vi "בדיקת מפל מתח בין הדקי הממסר תחת עומס bis5.vi"(8 "error":errorcluster, 10 "lines":tag="PXI1Slot8/port0/line1", 11 "Path for Log":path) -> (0 "error IO":errorcluster, 1 "בטוח כן/לא":bool, 2 "מפל מתח בין דקי הממסר תחת עומס":dbl, 3 "תוצאה זמנית":dbl)   [LabVIEW 2014]
uses:
  M9700 Driver/85/vi.lib/M9700 Modbus.llb/CTL Register Address.ctl
  M9700 Driver/86/vi.lib/M9700 Modbus.llb/CTL CMD Register.ctl
  <vilib>/Instr/_visa.llb/VISA Configure Serial Port (Instr).vi
  <vilib>/DAQmx/create/channels.llb/DAQmx Create Channel (DO-Digital Output).vi
  <vilib>/DAQmx/write.llb/DAQmx Write (Digital Bool 1Line 1Point).vi
panel:
  out "progress":dbl(slide) min=0.0 max=10.0 scale=0.0..10.0
  in  "stop":bool
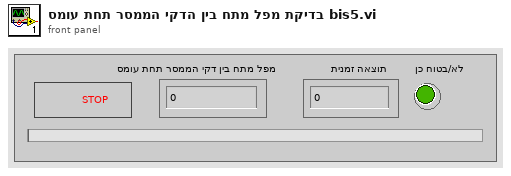
[diagram p1: front panel]
types:
  T1 = enum32{"Invalid", "Standard", "Closed", "Hidden", "Minimized", "Maximized"}
  T2 = typedef "CTL CMD Register.ctl" = u8
  T3 = typedef "CTL Register Address.ctl" = u16
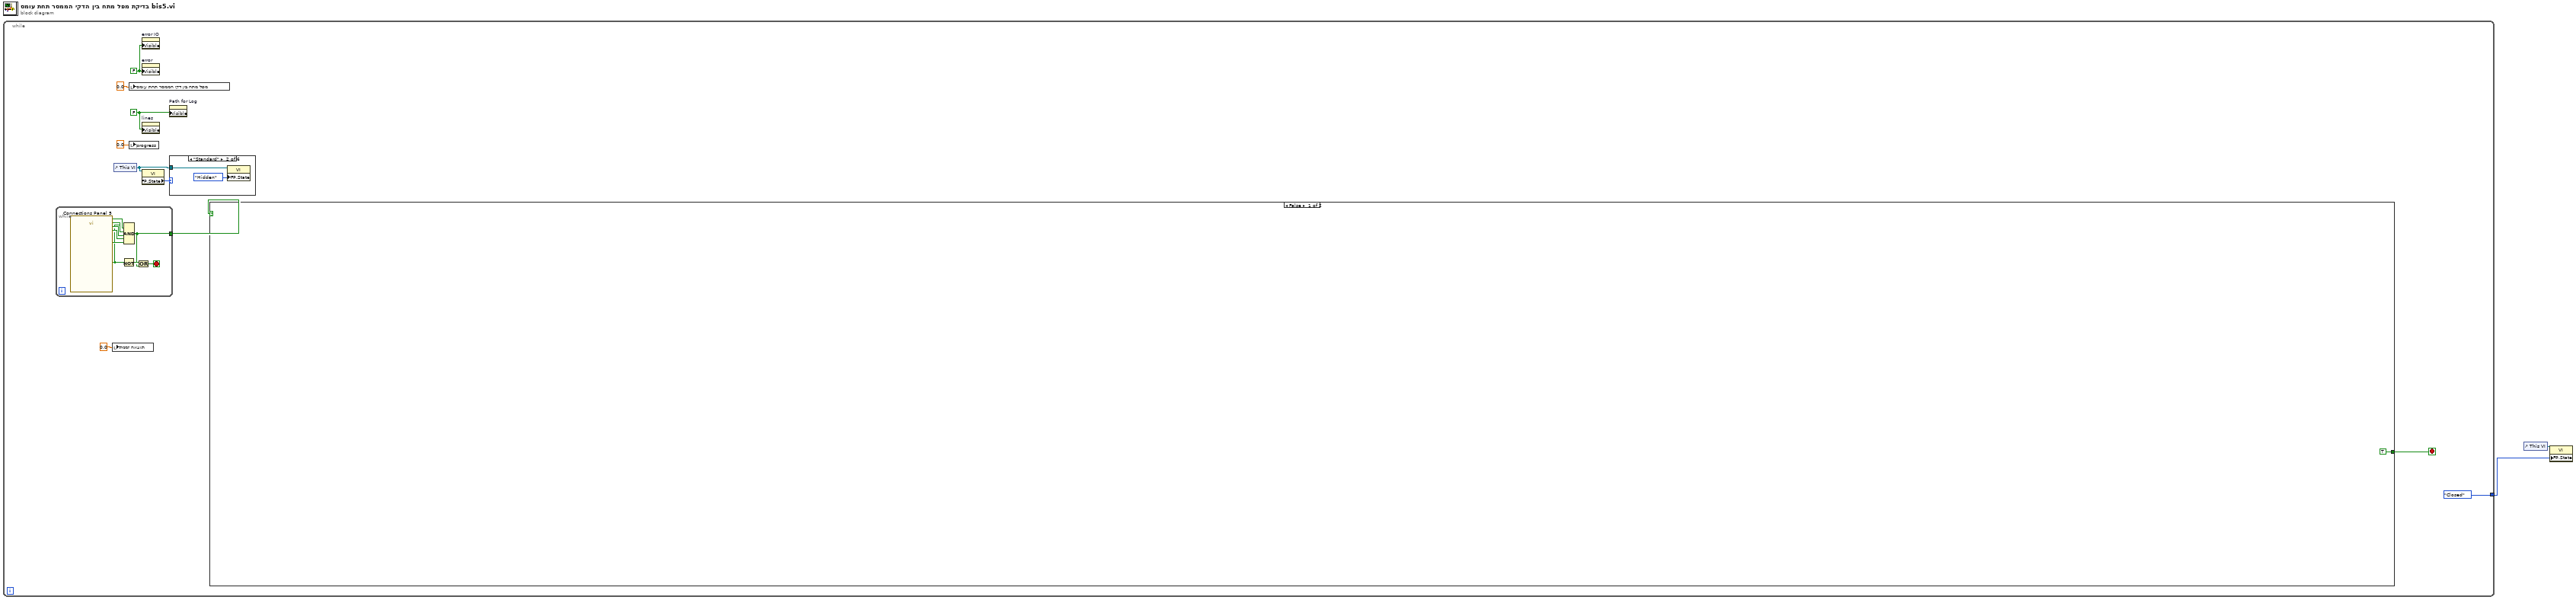
[diagram p0: block diagram]
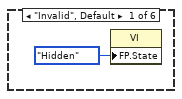
[diagram p2: hidden frame]
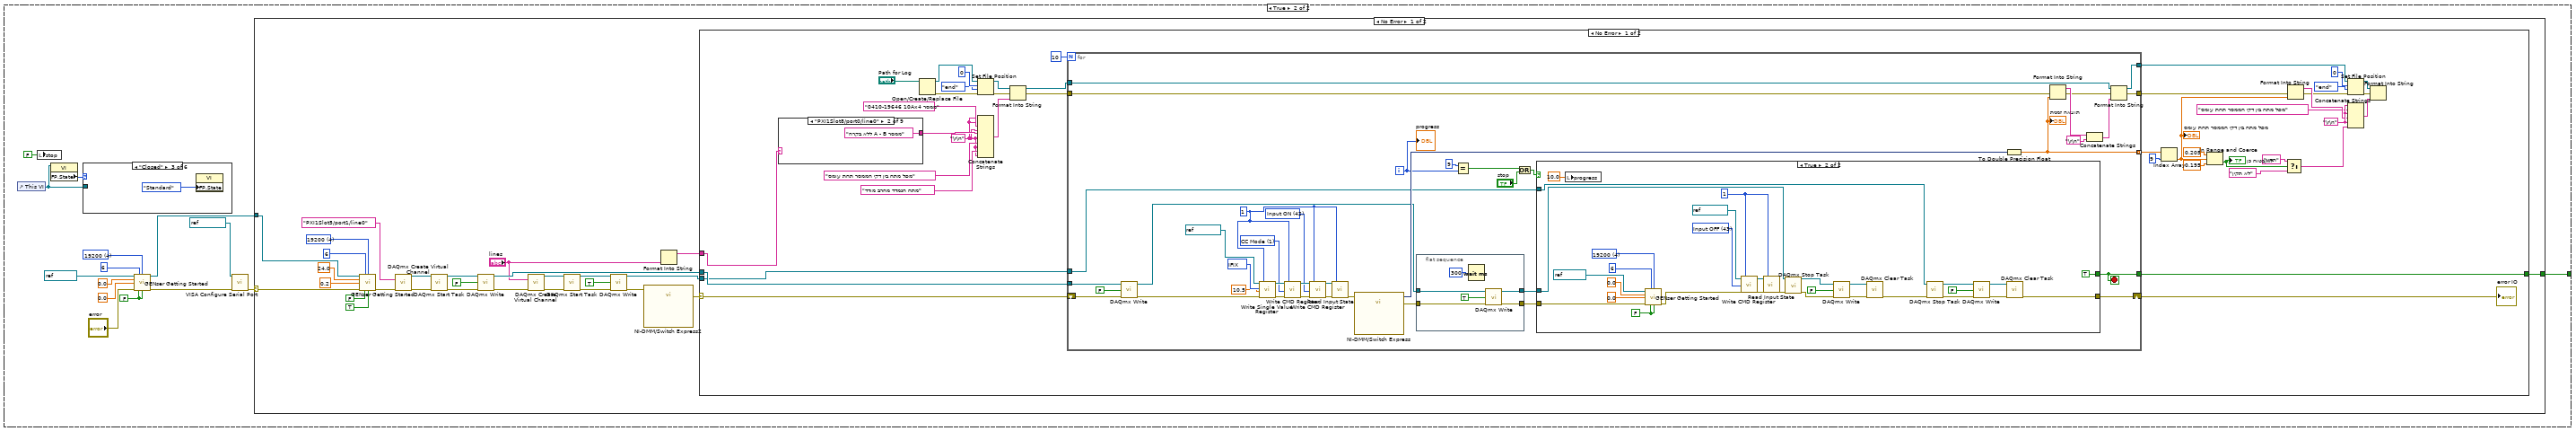
[diagram p7: hidden frame]
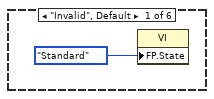
[diagram p8: hidden frame]
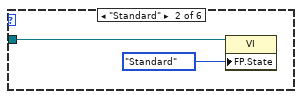
[diagram p9: hidden frame]
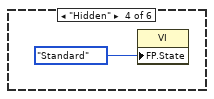
[diagram p10: hidden frame]
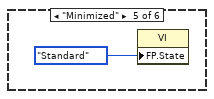
[diagram p11: hidden frame]
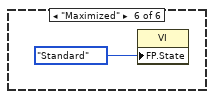
[diagram p12: hidden frame]
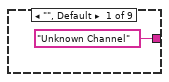
[diagram p13: hidden frame]
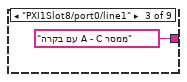
[diagram p14: hidden frame]
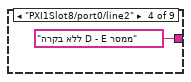
[diagram p15: hidden frame]
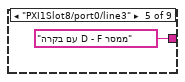
[diagram p16: hidden frame]
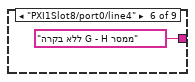
[diagram p17: hidden frame]
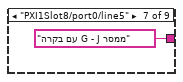
[diagram p18: hidden frame]
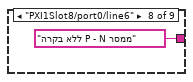
[diagram p19: hidden frame]
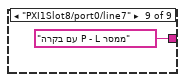
[diagram p20: hidden frame]
diagram:
  n1 = while {
    tunnel: [T1."Closed" ("Front Panel Window:State")] -> w1
    stop <- w12 stop-if-true
    w6 = FALSE ("Visible")
    w7 = FALSE ("Visible")
    n2 = while {
      tunnel: [w13] -> w11
      stop <- w16 stop-if-true
      n3 = call "Connections Panel 5.vi"() -> ("Input Name 10"=w17:bool, "Input Name 6"=w21:bool, "Input Name 7"=w20:bool, "Input Name 8"=w19:bool, "Input Name 9"=w18:bool, "OK"=w14:bool)  [unwired: 13 in, 1 out]
      n4 = Not(x=w14) -> (.not. x?=w15:bool)
      n5 = Compound Arithmetic op=AND(w14, w21, w20, w19, w18, w17) -> (w13:bool)
      n6 = Or(x=w15, y=w13) -> (x .or. y?=w16:bool)
    }
    n7 = local write "תוצאה זמנית"(0.0 ("תוצאה זמנית")) -> ()
    n8 = control-ref of="This VI"() -> (w5:refnum<vi>)
    n9 = local write "מפל מתח בין דקי הממסר תחת עומס"(0.0 ("מפל מתח בין דקי הממסר תחת עומס")) -> ()
    n10 = local write "progress"(0.0 ("progress")) -> ()
    n11 = property on="error IO" class="Clust (strict)"("Visible"=w7) -> ()  [unwired: 2 in, 2 out]
    n12 = property on="error" class="Clust (strict)"("Visible"=w7) -> ()  [unwired: 2 in, 2 out]
    n13 = property on="lines" class="DAQmxName"("Visible"=w6) -> ()  [unwired: 2 in, 2 out]
    n14 = property class="VI"(reference=w5) -> ("FP.State"=w4:T1)  [unwired: 1 in, 2 out]
    n15 = property on="Path for Log" class="Path"("Visible"=w6) -> ()  [unwired: 2 in, 2 out]
    n16 = case shown="\"Standard\"" w4 {
      tunnel: w5 -> [_ w23 _ _ _ _]
      frame "Invalid", Default {
        n17 = property class="VI"("FP.State"=T1."Hidden" ("Front Panel Window:State")) -> ()  [unwired: 2 in, 2 out]
      }
      frame "Standard" {
        n18 = property class="VI"(reference=w23, "FP.State"=T1."Hidden" ("Front Panel Window:State")) -> ()  [unwired: 1 in, 2 out]
      }
      frame "Closed" {
      }
      frame "Hidden" {
      }
      frame "Minimized" {
      }
      frame "Maximized" {
      }
    }
    n19 = case shown="False" w11 {
      tunnel: [TRUE w33] -> w12
      frame False {
      }
      frame True {
        w30 = FALSE ("Output On (T)")
        w37 = u16 4 items=["1200", "2400", "4800", "9600", "19200"] ("BAUD")
        n20 = control-ref of="This VI"() -> (w27:refnum<vi>)
        n21 = local write "stop"(FALSE ("stop")) -> ()
        n22 = property class="VI"(reference=w27) -> ("FP.State"=w28:T1)  [unwired: 1 in, 2 out]
        n23 = case shown="\"Closed\"" w28 {
          tunnel: w27 -> [_ w42 _ _ _ _]
          frame "Invalid", Default {
            n24 = property class="VI"("FP.State"=T1."Standard" ("Front Panel Window:State")) -> ()  [unwired: 2 in, 2 out]
          }
          frame "Standard" {
            n25 = property class="VI"(reference=w42, "FP.State"=T1."Standard" ("Front Panel Window:State")) -> ()  [unwired: 1 in, 2 out]
          }
          frame "Closed" {
            n26 = property class="VI"("FP.State"=T1."Standard" ("Front Panel Window:State")) -> ()  [unwired: 2 in, 2 out]
          }
          frame "Hidden" {
            n27 = property class="VI"("FP.State"=T1."Standard" ("Front Panel Window:State")) -> ()  [unwired: 2 in, 2 out]
          }
          frame "Minimized" {
            n28 = property class="VI"("FP.State"=T1."Standard" ("Front Panel Window:State")) -> ()  [unwired: 2 in, 2 out]
          }
          frame "Maximized" {
            n29 = property class="VI"("FP.State"=T1."Standard" ("Front Panel Window:State")) -> ()  [unwired: 2 in, 2 out]
          }
        }
        n30 = call "GENser Getting Started.vi"("VISA"=refnum<visa-resource-name> "COM6", "GEN Addr"=i16 6, "BAUD"=w37, "Voltage Limit"=0.0, "Current Limit"=0.0, "error"="error", "Reset (T)"=w30, "Output On (T)"=w30) -> ("VISA out"=w39:refnum<visa-resource-name>, "error out"=w26:errorcluster)  [unwired: 4 in, 2 out]
        n31 = call-poly "VISA Configure Serial Port"("VISA resource name"=refnum<visa-resource-name> "COM13", "error in (no error)"=w26) -> ("error out"=w31:errorcluster)  [unwired: 4 in, 9 out]
        n32 = case shown="No Error" w31 {
          selector: w31 -> [w73 _]
          tunnel: w39 -> [w75 _]
          tunnel: [w74 w209] -> w33
          frame No Error {
            w67 = u16 4 items=["1200", "2400", "4800", "9600", "19200"] ("BAUD")
            n33 = call "GENser Getting Started.vi"("VISA"=w75, "GEN Addr"=i16 6, "BAUD"=w67, "Voltage Limit"=24.0, "Current Limit"=0.2, "error"=w73, "Reset (T)"=FALSE, "Output On (T)"=TRUE) -> ("error out"=w61:errorcluster)  [unwired: 4 in, 3 out]
            n34 = call-poly <vilib>:"DAQmx Create Virtual Channel.vi"("lines"=tag "PXI1Slot5/port1/line0", "error in"=w61) -> ("task out"=w57:refnum<k21>, "error out"=w58:errorcluster)  [unwired: 12 in]
            n35 = call <vilib>:"DAQmx Start Task.vi"("task/channels in"=w57, "error in"=w58) -> ("task out"=w55:refnum<k21>, "error out"=w54:errorcluster)  [unwired: 12 in]
            n36 = call-poly <vilib>:"DAQmx Write.vi"("task/channels in"=w55, "data"=FALSE, "error in"=w54) -> ("task out"=w65:refnum<k21>, "error out"=w64:errorcluster)  [unwired: 10 in, 1 out]
            n37 = call-poly <vilib>:"DAQmx Create Virtual Channel.vi"("lines"="lines", "error in"=w64) -> ("task out"=w48:refnum<k21>, "error out"=w49:errorcluster)  [unwired: 12 in]
            n38 = call <vilib>:"DAQmx Start Task.vi"("task/channels in"=w48, "error in"=w49) -> ("task out"=w51:refnum<k21>, "error out"=w50:errorcluster)  [unwired: 12 in]
            n39 = call-poly <vilib>:"DAQmx Write.vi"("task/channels in"=w51, "data"=TRUE, "error in"=w50) -> ("task out"=w63:refnum<k21>, "error out"=w60:errorcluster)  [unwired: 10 in, 1 out]
            n40 = call "NI-DMM/Switch Express2"("error in"=w60) -> ("error out"=w59:errorcluster)  [unwired: 16 in, 2 out]
            n41 = Format Into String("lines") -> (resulting string=w66:string)  [unwired: 3 in, 1 out]
            n42 = case shown="No Error" w59 {
              selector: w59 -> [w117 _]
              tunnel: [w116 w204] -> w74
              tunnel: w65 -> [w115 _]
              tunnel: w66 -> [w114 _]
              tunnel: w63 -> [w113 _]
              frame No Error {
                w95 = "\r\n"
                w77 = "\r\n"
                n43 = case shown="\"PXI1Slot8/port0/line0\"" w114 {
                  tunnel: ["Unknown Channel" "ללא בקרה A - B ממסר" "עם בקרה A - C ממסר" "ללא בקרה D - E ממסר" "עם בקרה D - F ממסר" "ללא בקרה G - H ממסר" "עם בקרה G - J ממסר" "ללא בקרה P - N ממסר" "עם בקרה P - L ממסר"] -> w78
                  frame "", Default {
                  }
                  frame "PXI1Slot8/port0/line0" {
                  }
                  frame "PXI1Slot8/port0/line1" {
                  }
                  frame "PXI1Slot8/port0/line2" {
                  }
                  frame "PXI1Slot8/port0/line3" {
                  }
                  frame "PXI1Slot8/port0/line4" {
                  }
                  frame "PXI1Slot8/port0/line5" {
                  }
                  frame "PXI1Slot8/port0/line6" {
                  }
                  frame "PXI1Slot8/port0/line7" {
                  }
                }
                n44 = Open/Create/Replace File(file path (use dialog)="Path for Log") -> (refnum out=w105:refnum<file>, error out=w104:errorcluster)  [unwired: 5 in, 1 out]
                n45 = Set File Position(offset (in bytes) (0)=i64 0, refnum=w105, from (0:start)=enum16{"start", "end", "current"}."end", error in=w104) -> (refnum out=w101:refnum<file>, error out=w98:errorcluster)
                n46 = Concatenate Strings(w77, w77, "0410-19646 10Ax4 ממסר", w77, w78, w77, "מפל מתח בין דקי הממסר תחת עומס", w77, "מתח הנמדד מהרב מודד", w77) -> (w103:string)
                n47 = Format Into String(initial string=w101, error in=w98, w103) -> (resulting string=w96:refnum<file>, error out=w97:errorcluster)  [unwired: 1 in]
                n48 = for {
                  N: 10 -> [_]
                  tunnel: [w148] -> w116
                  shift-right: [w146] -> w76
                  shift-left: w117 -> [w141]
                  tunnel: [w128] -> w111 mode=indexing
                  tunnel: w115 -> [w142]
                  tunnel: w97 -> [w132]
                  tunnel: w96 -> [w134]
                  tunnel: [w131] -> w89
                  tunnel: [w130] -> w80
                  tunnel: w113 -> [w129]
                  i -> [w145]
                  stop <- w148 stop-if-true
                  w156 = T2 42 items=["CC Mode"=1, "CV Mode"=2, "CW Mode"=3, "CR Mode"=4, "Short Mode"=26, "Set SysPara"=41, "Input ON"=42, "Input OFF"=43] ("CMD Register Value")
                  w159 = u8 1 ("Load Address")
                  w162 = T2 1 items=["CC Mode"=1, "CV Mode"=2, "CW Mode"=3, "CR Mode"=4, "Short Mode"=26, "Set SysPara"=41, "Input ON"=42, "Input OFF"=43] ("CMD Register Value")
                  w165 = T3 2561 items=["REMOTE"=1283, "ISTATE"=1296, "CMD"=2560, "IFIX"=2561, "UFIX"=2563, "PFIX"=2565, "RFIX"=2567, "IMAX"=2612, "UMAX"=2614, "PMAX"=2616, "U"=2816, "I"=2818, "MODEL"=2822, "EDITION"=2823] ("Register Address")
                  n49 = call-poly <vilib>:"DAQmx Write.vi"("task/channels in"=w142, "data"=FALSE, "error in"=w141) -> ("task out"=w140:refnum<k21>, "error out"=w127:errorcluster)  [unwired: 10 in, 1 out]
                  n50 = call "Write Single Value Register.vi"("VISA resource name"=refnum<visa-resource-name> "COM13", "Starting Address(HEX)"=w165, "Register Single Value"=sgl 10.5, "error in"=w127, "Load Address"=w159) -> ("VISA resource name out"=w164:refnum<visa-resource-name>, "error out"=w163:errorcluster)  [unwired: 13 out]
                  n51 = call "Write CMD Register.vi"("VISA resource name"=w164, "CMD Value"=w162, "error in"=w163, "Load Address"=w159) -> ("VISA resource name out"=w160:refnum<visa-resource-name>, "error out"=w157:errorcluster)  [unwired: 14 out]
                  n52 = call "Write CMD Register.vi"("VISA resource name"=w160, "CMD Value"=w156, "error in"=w157, "Load Address"=w159) -> ("VISA resource name out"=w158:refnum<visa-resource-name>, "error out"=w155:errorcluster)  [unwired: 14 out]
                  n53 = call "Read Input State.vi"("VISA resource name"=w158, "error in"=w155, "Load Address"=w159) -> ("error out"=w154:errorcluster)  [unwired: 16 out]
                  n54 = call "NI-DMM/Switch Express"("error in"=w154) -> ("signals out"=w153:dynamicdata, "error out"=w143:errorcluster)  [unwired: 16 in, 1 out]
                  n55 = flat-sequence {
                    tunnel: [w171] -> w144
                    tunnel: w143 -> [w170]
                    tunnel: w140 -> [w168]
                    tunnel: [w167] -> w138
                    frame #0 {
                      n56 = Wait (ms)(milliseconds to wait=u32 300) -> ()  [unwired: 1 out]
                      n57 = call-poly <vilib>:"DAQmx Write.vi"("task/channels in"=w168, "data"=TRUE, "error in"=w170) -> ("task out"=w167:refnum<k21>, "error out"=w171:errorcluster)  [unwired: 10 in, 1 out]
                    }
                  }
                  n58 = Equal?(x=9, y=w145) -> (x = y?=w150:bool)
                  n59 = Or(x=w150, y="stop") -> (x .or. y?=w151:bool)
                  n60 = case shown="True" w151 {
                    tunnel: [FALSE TRUE] -> w148
                    tunnel: w144 -> [w172 w197]
                    tunnel: [w172 w177] -> w146
                    tunnel: w138 -> [_ w183]
                    tunnel: w129 -> [_ w175]
                    frame False {
                    }
                    frame True {
                      w191 = u8 1 ("Load Address")
                      w194 = T2 43 items=["CC Mode"=1, "CV Mode"=2, "CW Mode"=3, "CR Mode"=4, "Short Mode"=26, "Set SysPara"=41, "Input ON"=42, "Input OFF"=43] ("CMD Register Value")
                      w196 = FALSE ("Reset (T)")
                      w199 = u16 4 items=["1200", "2400", "4800", "9600", "19200"] ("BAUD")
                      n61 = local write "progress"(10.0 ("progress")) -> ()
                      n62 = call "GENser Getting Started.vi"("VISA"=refnum<visa-resource-name> "COM6", "GEN Addr"=i16 6, "BAUD"=w199, "Voltage Limit"=0.0, "Current Limit"=0.0, "error"=w197, "Reset (T)"=w196, "Output On (T)"=w196) -> ("error out"=w174:errorcluster)  [unwired: 4 in, 3 out]
                      n63 = call "Write CMD Register.vi"("VISA resource name"=refnum<visa-resource-name> "COM13", "CMD Value"=w194, "error in"=w174, "Load Address"=w191) -> ("VISA resource name out"=w192:refnum<visa-resource-name>, "error out"=w195:errorcluster)  [unwired: 14 out]
                      n64 = call "Read Input State.vi"("VISA resource name"=w192, "error in"=w195, "Load Address"=w191) -> ("error out"=w184:errorcluster)  [unwired: 16 out]
                      n65 = call <vilib>:"DAQmx Stop Task.vi"("task/channels in"=w183, "error in"=w184) -> ("task out"=w189:refnum<k21>, "error out"=w187:errorcluster)  [unwired: 12 in]
                      n66 = call-poly <vilib>:"DAQmx Write.vi"("task/channels in"=w189, "data"=FALSE, "error in"=w187) -> ("task out"=w186:refnum<k21>, "error out"=w185:errorcluster)  [unwired: 10 in, 1 out]
                      n67 = call <vilib>:"DAQmx Clear Task.vi"("task in"=w186, "error in"=w185) -> ("error out"=w176:errorcluster)  [unwired: 13 in]
                      n68 = call <vilib>:"DAQmx Stop Task.vi"("task/channels in"=w175, "error in"=w176) -> ("task out"=w182:refnum<k21>, "error out"=w180:errorcluster)  [unwired: 12 in]
                      n69 = call-poly <vilib>:"DAQmx Write.vi"("task/channels in"=w182, "data"=FALSE, "error in"=w180) -> ("task out"=w179:refnum<k21>, "error out"=w178:errorcluster)  [unwired: 10 in, 1 out]
                      n70 = call <vilib>:"DAQmx Clear Task.vi"("task in"=w179, "error in"=w178) -> ("error out"=w177:errorcluster)  [unwired: 13 in]
                    }
                  }
                  n71 = To Double Precision Float(number=w153) -> (double precision float=w128:dbl)
                  "תוצאה זמנית" <- w128
                  n72 = Format Into String(error in=w132, w128) -> (resulting string=w136:string, error out=w133:errorcluster)  [unwired: 2 in]
                  n73 = Concatenate Strings(w136, "\r\n") -> (w135:string)
                  n74 = Format Into String(initial string=w134, error in=w133, w135) -> (resulting string=w131:refnum<file>, error out=w130:errorcluster)  [unwired: 1 in]
                  "progress" <- w145
                }
                "error IO" <- w76
                n75 = Index Array(array=w111, index=9) -> (element=w88:dbl)
                "מפל מתח בין דקי הממסר תחת עומס" <- w88
                n76 = In Range and Coerce(upper limit=0.205, x=w88, lower limit=0.195) -> (In Range?=w83:bool)  [unwired: 1 out]
                "בטוח כן/לא" <- w83
                n77 = Select(t="תקין", s=w83, f="לא תקין") -> (s? t:f=w82:string)
                n78 = Format Into String(error in=w80, w88) -> (resulting string=w87:string, error out=w81:errorcluster)  [unwired: 2 in]
                n79 = Set File Position(offset (in bytes) (0)=i64 0, refnum=w89, from (0:start)=enum16{"start", "end", "current"}."end", error in=w81) -> (refnum out=w92:refnum<file>, error out=w91:errorcluster)
                n80 = Concatenate Strings(w95, "מפל מתח בין דקי הממסר תחת עומס" ("string"), w95, w87, w95, w82) -> (w90:string)
                n81 = Format Into String(initial string=w92, error in=w91, w90) -> ()  [unwired: 1 in, 2 out]
              }
              frame Error {
                n82 = Two Button Dialog(message="בעיית דגימת נתונים ע\"י הכרטיס רב מודד", 1:"ביטול" ("F button name (\"Cancel\")"), 2:"נסה שוב" ("T button name (\"OK\")")) -> (T button?=w205:bool)
                n83 = Not(x=w205) -> (.not. x?=w204:bool)
              }
            }
          }
          frame Error {
            n84 = Two Button Dialog(message="בעיית תקשורת עם ספק קוח", 1:"ביטול" ("F button name (\"Cancel\")"), 2:"נסה שוב" ("T button name (\"OK\")")) -> (T button?=w210:bool)
            n85 = Not(x=w210) -> (.not. x?=w209:bool)
          }
        }
      }
    }
  }
  n86 = control-ref of="This VI"() -> (w2:refnum<vi>)
  n87 = property class="VI"(reference=w2, "FP.State"=w1) -> ()  [unwired: 1 in, 2 out]
